vi "Daten speichern auf PC.vi"(4 "Password":string="iag", 6 "User Name":string="iag", 7 "IP Adresse":string, 8 "error in":errorcluster, 9 "Pfad PLC":string, 10 "Dateinamen":string[](array[string]), 11 "Pfad PC":path caption="Lokaler Pfad") -> (0 "error out":errorcluster, 2 "ohne Fehler":bool, 3 "Dateipfad out":path[](array[path]))   [LabVIEW 2020, in "FTP WebDAV.lvlib"]
doc: "Speichert ein Array von Dateinamen von der cRIO auf den PC.\nftp ode webDAV (je nach FGV FTP WebDAV.vi Ausgang).\n\nSowohl für webDAV als auch ftp genügt diese URL/Pfad Notation:\nhome/lvuser/natinst/bin/ oder c/KonfigIAG/\n(vorne kein / notwendig, hinten schon ! - ftp ist das egal, bei webDAV wird http://IP/files/ intern voran gestellt)\n\nriw - 2019-02-22"
uses:
  FTP WebDAV.lvlib
  Aktionen FTP WebDAV.ctl
  <vilib>/WebDAVClient/Simple Get File.vi
  <vilib>/FTP/NI_FTP.lvlib
  <vilib>/WebDAVClient/NI_WebDAV.lvlib
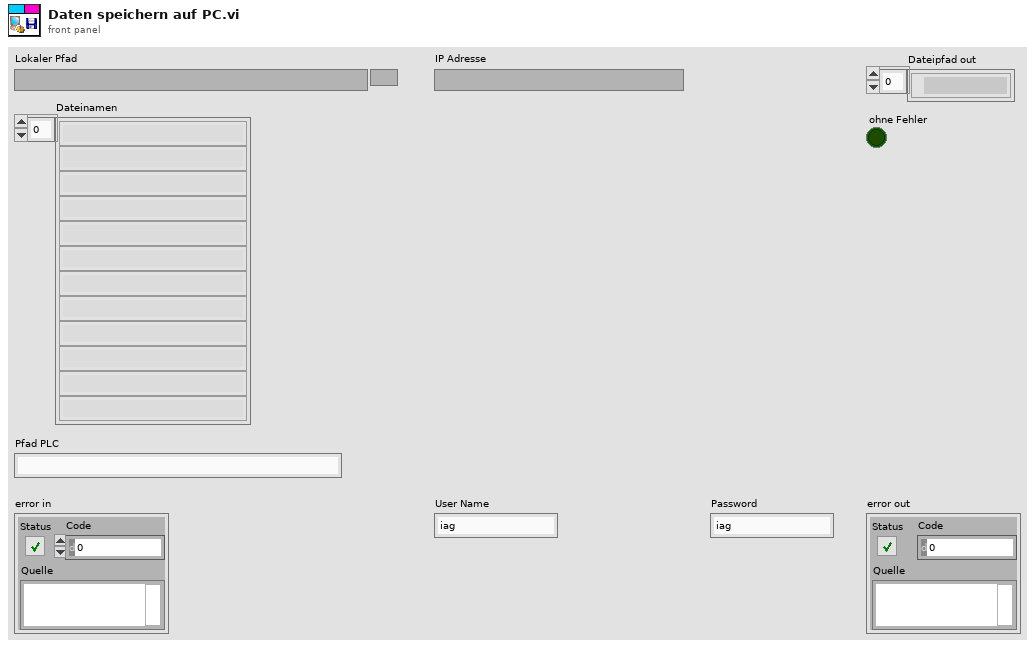
[diagram p1: front panel]
types:
  T1 = typedef "FTP WebDAV.lvlib/Aktionen FTP WebDAV.ctl" = enum16{"lesen", "erkennen"}
  T2 = typedef "FTP WebDAV.lvlib/Enum FTP WebDAV.ctl" = enum16{" nix", "ftp", "webDAV"}
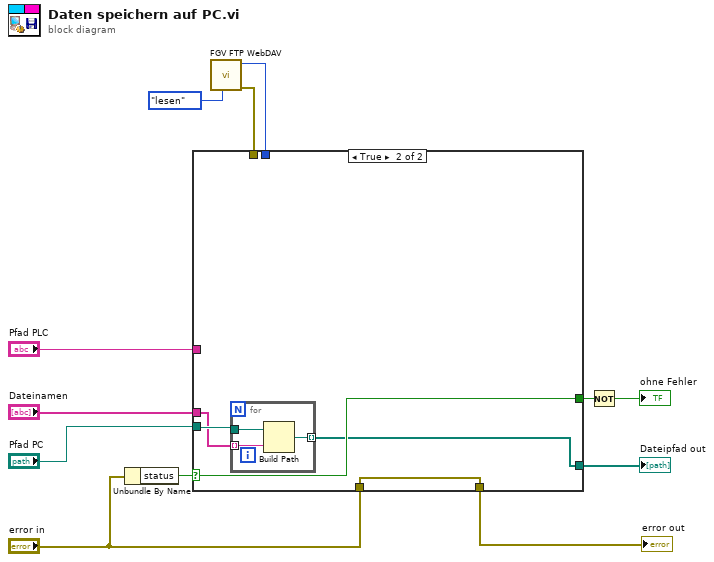
[diagram p0: block diagram]
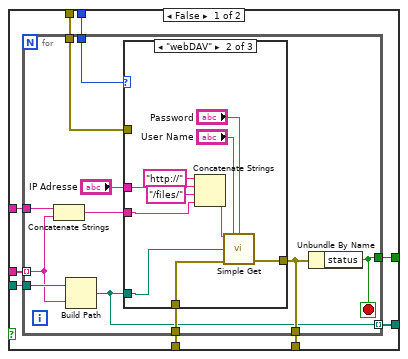
[diagram p2: hidden frame]
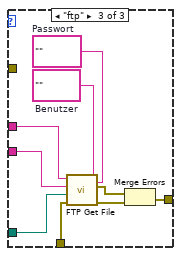
[diagram p4: hidden frame]
diagram:
  n1 = Unbundle By Name("error in") -> ("status"=w9:bool)
  n2 = call "FGV FTP WebDAV.vi"("Aktionen"=Aktionen_FTP_WebDAV."lesen") -> ("Fehler (Ausgang)"=w4:errorcluster, "ftp webDAV"=w2:T2)  [unwired: 6 in, 3 out]
  n3 = case shown="True" w9 {
    selector: w9 -> [_ w56]
    tunnel: "Dateinamen" -> [w21 w54]
    tunnel: "Pfad PLC" -> [w20 _]
    tunnel: "Pfad PC" -> [w19 w55]
    tunnel: [w18 w57] -> w8
    tunnel: [w16 w56] -> w7
    tunnel: "error in" -> [w17 w57]
    tunnel: w2 -> [w15 _]
    tunnel: w4 -> [w14 _]
    tunnel: [w13 w53] -> w1
    frame False {
      n4 = for {
        tunnel: w19 -> [w30]
        tunnel: w20 -> [w32]
        tunnel: w21 -> [w29] mode=indexing
        tunnel: [w26] -> w16
        tunnel: w17 -> [w28]
        tunnel: [w27] -> w18
        tunnel: w15 -> [w24]
        tunnel: w14 -> [w23]
        tunnel: [w22] -> w13 mode=indexing
        stop <- w26 stop-if-true
        n5 = Concatenate Strings(w32, w29) -> (w31:string)
        n6 = Build Path(base path=w30, name or relative path=w29) -> (appended path=w22:path)
        n7 = case shown="\"webDAV\"" w24 {
          tunnel: w31 -> [_ w43 w52]
          tunnel: w22 -> [_ w42 w51]
          tunnel: w28 -> [_ w41 w50]
          tunnel: [w33 w40 w49] -> w27
          tunnel: "IP Adresse" -> [_ w39 w48]
          tunnel: w23 -> [w33 _ _]
          frame " nix", Default {
          }
          frame "webDAV" {
            n8 = Concatenate Strings("http://" ("String"), w39, "/files/" ("String"), w43) -> (w36:string)
            n9 = call-poly <vilib>:"Simple Get.vi"("remote file uri"=w36, "username"="User Name", "password"="Password", "local file path"=w42, "error in (no error)"=w41) -> ("error out"=w40:errorcluster)  [unwired: 9 in, 1 out]
          }
          frame "ftp" {
            w46 = ""  # Passwort
            w47 = ""  # Benutzer
            n10 = call <vilib>:"FTP Get File.vi"("password"=w46, "user"=w47, "error in (no error)"=w50, "local path"=w51, "remote path"=w52, "host"=w48) -> ("error out"=w45:errorcluster, "file error"=w44:errorcluster)  [unwired: 4 in]
            n11 = Merge Errors(w44, w45) -> (w49:errorcluster)
          }
        }
        n12 = Unbundle By Name(w27) -> ("status"=w26:bool)
      }
    }
    frame True {
      n13 = for {
        tunnel: w55 -> [w60]
        tunnel: w54 -> [w59] mode=indexing
        tunnel: [w58] -> w53 mode=indexing
        n14 = Build Path(base path=w60, name or relative path=w59) -> (appended path=w58:path)
      }
    }
  }
  "error out" <- w8
  "Dateipfad out" <- w1
  n15 = Not(x=w7) -> (.not. x?=→"ohne Fehler":bool)
